vi "OnlineData_HandleDVR.vi"(8 "error in":errorcluster, 11 "func":T1) -> (0 "error out":errorcluster, 3 "DVR_OUT":refnum<data-value>)   [LabVIEW 2018, in "MonSys_Server_Actor.lvlib" / "MonSys_Server_Actor.lvclass"]
doc: "Handle a SystemState DVR here"
uses:
  MonSys_Server_Actor.lvclass
  typedefs/OnlineData_HandleDVR_func.ctl
  _MonSys_LIB/OnlineData.ctl
  _MonSys_LIB/OnlineData_State.ctl
  _MonSys_LIB/_MonSys_LIB.lvlib
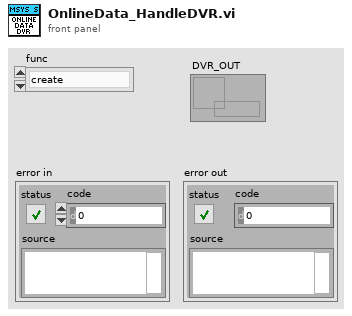
[diagram p1: front panel]
types:
  T1 = typedef "OnlineData_HandleDVR_func.ctl" = enum16{"create", "get", "close"}
  T2 = typedef "_MonSys_LIB.lvlib/OnlineData.ctl" = cluster{"Online":bool, "Info":string, "OnlineData_State":T3}
  T3 = typedef "_MonSys_LIB.lvlib/OnlineData_State.ctl" = u16
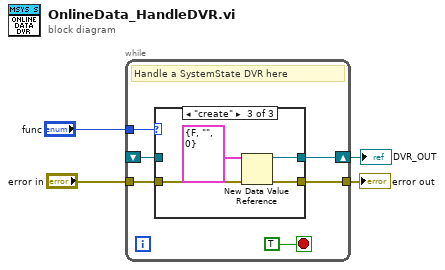
[diagram p0: block diagram]
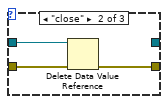
[diagram p3: hidden frame]
diagram:
  n1 = while {
    tunnel: "func" -> [w10]
    shift-right: [w9] -> w1
    shift-left: _ -> [w6]
    tunnel: "error in" -> [w5]
    tunnel: [w7] -> w3
    stop <- TRUE stop-if-true
    # "Handle a SystemState DVR here"
    n2 = case shown="\"create\"" w10 {
      tunnel: [w11 _ w19] -> w9
      tunnel: [w12 w13 w18] -> w7
      tunnel: w5 -> [w12 w14 w17]
      tunnel: w6 -> [w11 w15 _]
      frame "get", Default {
      }
      frame "close" {
        n3 = Delete Data Value Reference(data value reference=w15, error in=w14) -> (error out=w13:errorcluster)  [unwired: 1 out]
      }
      frame "create" {
        n4 = New Data Value Reference(data value=T2 {"Online"=FALSE, "Info"="", "OnlineData_State"=0} ("Data"), error in=w17) -> (data value reference=w19:refnum<data-value>, error out=w18:errorcluster)
      }
    }
  }
  "error out" <- w3
  "DVR_OUT" <- w1
